vi "String to Word.vi"(10 "Byte Order (0:big-endian, network order)":T1(ring), 11 "String":string) -> (2 "Int16 Data":i16[](array[numeric]))   [LabVIEW 2020, in "Agilent 90000 Series.lvlib"]
doc: "Converts the stings to Int16 data."
uses:
  Agilent 90000 Series.lvlib
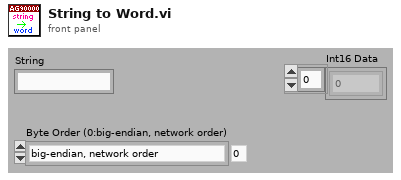
[diagram p1: front panel]
types:
  T1 = enum16{"big-endian, network order", "native, host order", "little-endian"}
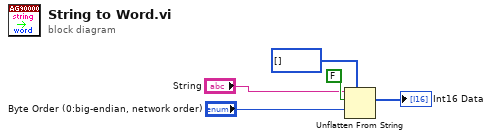
[diagram p0: block diagram]
diagram:
  n1 = Unflatten From String(type=i16[] [], binary string="String", data includes array or string size? (T)=FALSE, byte order (0:big-endian, network order)="Byte Order (0:big-endian, network order)") -> (value=→"Int16 Data":i16[])  [unwired: 1 in, 2 out]
